vi "74_Vision_RC Servo_DC_Moto_2.vi"() -> ()   [LabVIEW 2018]
uses:
  <userlib>/KNR OS 4.0 LabVIEW Toolkit/Type Definition/Resource.ctl
  <userlib>/KNR OS 4.0 LabVIEW Toolkit/Type Definition/RC Servo Port.ctl
  <userlib>/KNR OS 4.0 LabVIEW Toolkit/Type Definition/DC Motor Port.ctl
panel:
  out "area":dbl
  out "RC Pulse Width (uS)":u16[](array[numeric])
  out "Image Out":T1(plugin-control)
  in  "stop":bool
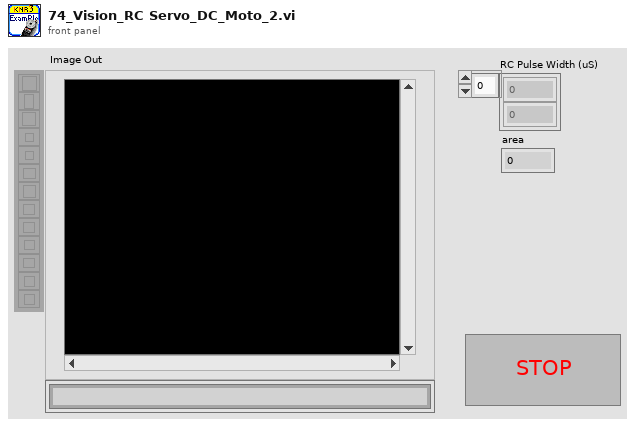
[diagram p1: front panel]
types:
  T1 = typedef "IMAQ Image.ctl" = refnum<image>
  T2 = typedef "DC Motor Port.ctl" = u16
  T3 = typedef "RC Servo Port.ctl" = u16
  T4 = typedef "Resource.ctl" = enum16{"KNRm_DDRC", "KNRm_DDDD", "KNRm_DDDR", "KNRm_DDDC", "KNR", "KNRm_neww"}
  T5 = typedef "KNR3 Reference.ctl" = cluster{"FPGA Session":refnum<class "FPGA Interface Base.lvclass">, "Resource":T4}
  T6 = cluster{"Left":dbl, "Top":dbl, "Right":dbl, "Bottom":dbl}
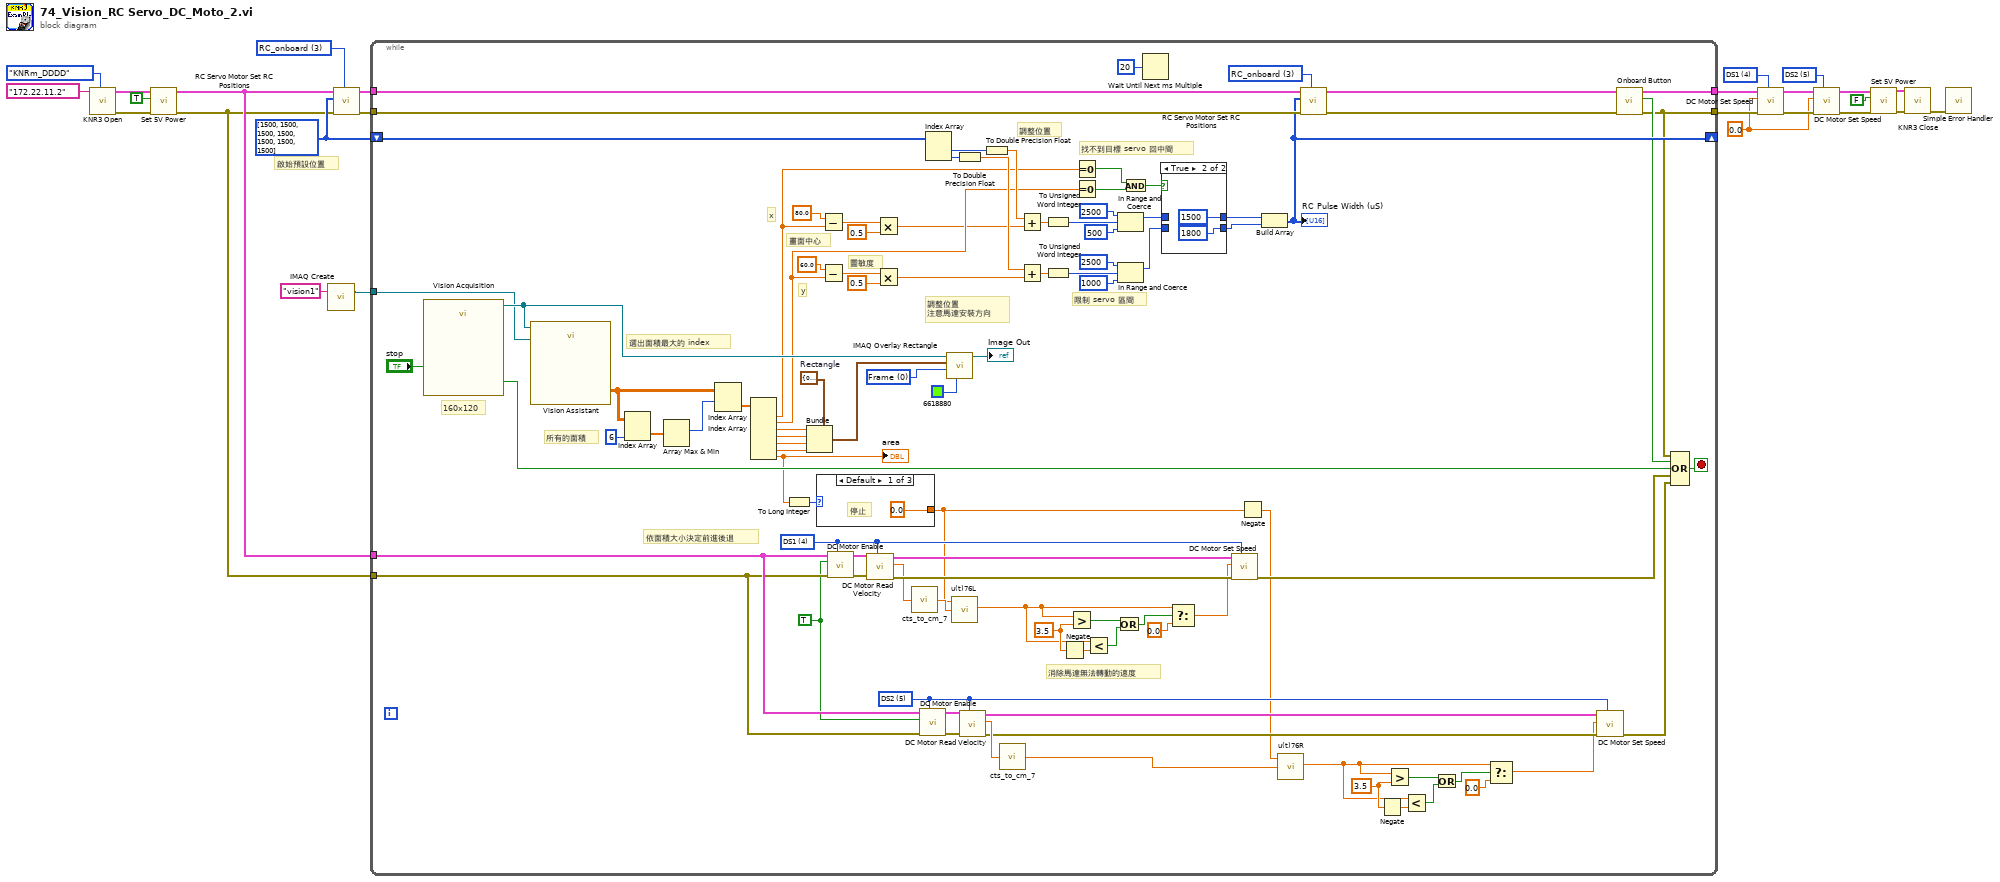
[diagram p0: block diagram]
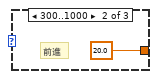
[diagram p2: hidden frame]
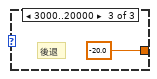
[diagram p3: hidden frame]
diagram:
  w1 = T2 5 items=["DS1"=4, "DS2"=5, "DS3"=6, "DS4"=7] ("Port (DS1)")
  w2 = T2 4 items=["DS1"=4, "DS2"=5, "DS3"=6, "DS4"=7] ("Port (DS1)")
  w3 = 0.0 ("Speed (+-100%)")
  w13 = u16[] [1500, 1500, 1500, 1500, 1500, 1500, 1500] ("RC Pulse Width (1500 uS)")
  w16 = T3 3 items=["RC_onboard"=3, "RC_box"=9] ("Port (RC_onboard)")
  # "啟始預設位置"
  n1 = call <userlib>:"KNR3 Open.vi"("Resource"=Resource."KNRm_DDDD", "IP"="172.22.11.2") -> ("error out"=w22:errorcluster, "KNR out"=w23:T5)  [unwired: 8 in]
  n2 = call <userlib>:"Set 5V Power.vi"("error in (no error)"=w22, "5V Power(T)"=TRUE ("5V Power"), "KNR in"=w23) -> ("error out"=w11:errorcluster, "KNR out"=w12:T5)  [unwired: 7 in]
  n3 = call "IMAQ Create"("Image Name"="vision1") -> ("New Image"=w14:T1)  [unwired: 4 in, 1 out]
  n4 = call <userlib>:"RC Servo Motor Set RC Positions.vi"("Port (RC_onboard)"=w16, "RC Pulse Width (1500 uS)"=w13, "KNR in"=w12) -> ("KNR out"=w17:T5)  [unwired: 7 in, 1 out]
  n5 = while {
    tunnel: w17 -> [w120]
    tunnel: [w43] -> w10
    tunnel: w11 -> [w118]
    tunnel: [w41] -> w9
    tunnel: w14 -> [w100]
    shift-right: [w84] -> _
    shift-left: w13 -> [w87]
    tunnel: w12 -> [w50]
    tunnel: w11 -> [w49]
    stop <- w117 stop-if-true
    w28 = 3.5
    w36 = 3.5
    w47 = u32 0 items=["Frame", "Fill", "Highlight"] ("Drawing Mode (Frame)")
    w53 = T2 5 items=["DS1"=4, "DS2"=5, "DS3"=6, "DS4"=7] ("Port 2")
    w44 = TRUE ("Enable Motor(F)")
    w66 = T2 4 items=["DS1"=4, "DS2"=5, "DS3"=6, "DS4"=7] ("Port 2")
    w113 = T6 {"Left"=0.0, "Top"=0.0, "Right"=0.0, "Bottom"=0.0}  # Rectangle
    w115 = T3 3 items=["RC_onboard"=3, "RC_box"=9] ("RC Motor")
    # "調整位置\n注意馬達安裝方向"
    # "依面積大小決定前進後退"
    # "消除馬達無法轉動的速度"
    # "調整位置"
    # "靈敏度"
    # "所有的面積"
    # "畫面中心"
    # "限制 servo 區間"
    # "找不到目標 servo 回中間"
    # "y"
    # "x"
    # "160x120"
    # "選出面積最大的 index"
    n6 = call "Vision Acquisition"("Stop (F)"="stop") -> ("Image Out"=w105:T1, "Stopped"=w98:bool)  [unwired: 24 in, 1 out]
    n7 = call "Vision Assistant"("Image In"=w105, "Image Dst"=w100) -> ("Particle Measurements (Pixels) (Particle Analysis 1)"=w104:dbl[][])  [unwired: 22 in, 3 out]
    n8 = Index Array "Index Array"(array=w104, index (col)=6 ("disabled index (col)")) -> (element=w103:dbl[])  [unwired: 1 in]
    n9 = Array Max & Min(array=w103) -> (max index (indices)=w102:i32)  [unwired: 3 out]
    n10 = Index Array "Index Array"(array=w104, index (row)=w102) -> (element=w114:dbl[])  [unwired: 1 in]
    n11 = Index Array "Index Array"(array=w114) -> (element #1=w77:dbl, element #2=w76:dbl, element #3=w112:dbl, element #4=w111:dbl, element #5=w110:dbl, element #6=w109:dbl, element #7=w60:dbl)  [unwired: 7 in]
    "area" <- w60
    n12 = To Long Integer(number=w60) -> (32bit integer=w46:i32)
    n13 = Bundle "Bundle"(cluster=w113, "Left"=w112, "Top"=w111, "Right"=w110, "Bottom"=w109) -> (w108:T6)
    n14 = case shown="Default" w46 {
      tunnel: [0.0 20.0 -20.0] -> w40
      frame Default {
        # "停止"
      }
      frame 300..1000 {
        # "前進"
      }
      frame 3000..20000 {
        # "後退"
      }
    }
    n15 = Subtract(x=80.0 ("y"), y=w77) -> (x-y=w94:dbl)
    n16 = Subtract(x=60.0 ("y"), y=w76) -> (x-y=w95:dbl)
    n17 = call <userlib>:"DC Motor Enable.vi"("Port (DS1)"=w66, "error in (no error)"=w49, "Enable Motor(F)"=w44, "KNR in"=w50) -> ("error out"=w62:errorcluster, "KNR out"=w61:T5)  [unwired: 6 in]
    n18 = call <userlib>:"DC Motor Read Velocity.vi"("Port (DS1)"=w66, "error in (no error)"=w62, "KNR in"=w61) -> ("error out"=w65:errorcluster, "Velocity (cts/sec)"=w63:dbl, "KNR out"=w64:T5)  [unwired: 6 in]
    n19 = Multiply(x=w94, y=0.5) -> (x*y=w75:dbl)
    n20 = Multiply(x=w95, y=0.5) -> (x*y=w74:dbl)
    n21 = call "cts_to_cm_7.vi"("cts"=w63) -> ("cm"=w45:dbl)
    n22 = call <userlib>:"DC Motor Enable.vi"("Port (DS1)"=w53, "error in (no error)"=w49, "Enable Motor(F)"=w44, "KNR in"=w50) -> ("error out"=w57:errorcluster, "KNR out"=w58:T5)  [unwired: 6 in]
    n23 = Index Array "Index Array"(array=w87) -> (element #1=w86:u16, element #2=w85:u16)  [unwired: 2 in]
    n24 = call "IMAQ Overlay Rectangle"("Color"=u32 6618880, "Drawing Mode (Frame)"=w47, "Rectangle"=w108, "Image"=w105) -> ("Image Out"=→"Image Out":T1)  [unwired: 6 in, 1 out]
    n25 = call "u(t)76L.vi"("Velocity"=w45, "Desire Velosity"=w40) -> ("u(t)"=w34:dbl)  [unwired: 6 in]
    n26 = To Double Precision Float(number=w85) -> (double precision float=w78:dbl)
    n27 = call <userlib>:"DC Motor Read Velocity.vi"("Port (DS1)"=w53, "error in (no error)"=w57, "KNR in"=w58) -> ("error out"=w54:errorcluster, "Velocity (cts/sec)"=w56:dbl, "KNR out"=w55:T5)  [unwired: 6 in]
    n28 = To Double Precision Float(number=w86) -> (double precision float=w79:dbl)
    n29 = call "cts_to_cm_7.vi"("cts"=w56) -> ("cm"=w59:dbl)
    n30 = Add(x=w79, y=w75) -> (x+y=w96:dbl)
    n31 = Add(x=w78, y=w74) -> (x+y=w97:dbl)
    n32 = To Unsigned Word Integer(number=w96) -> (unsigned 16bit integer=w81:u16)
    n33 = To Unsigned Word Integer(number=w97) -> (unsigned 16bit integer=w80:u16)
    n34 = Negate(x=w36) -> (-x=w35:dbl)
    n35 = Greater?(x=w34, y=w36) -> (0:w33:bool)
    n36 = Equal To 0?(x=w77) -> (x = 0?=w71:bool)
    n37 = Equal To 0?(x=w76) -> (x = 0?=w72:bool)
    n38 = Less?(x=w34, y=w35) -> (x < y?=w32:bool)
    n39 = Or(x=w33, y=w32) -> (x .or. y?=w37:bool)
    n40 = In Range and Coerce(upper limit=u16 2500, x=w81, lower limit=u16 500) -> (coerced(x)=w70:u16)  [unwired: 1 out]
    n41 = In Range and Coerce(upper limit=u16 2500, x=w80, lower limit=u16 1000) -> (coerced(x)=w69:u16)  [unwired: 1 out]
    n42 = And(x=w71, y=w72) -> (x .and. y?=w73:bool)
    n43 = Wait Until Next ms Multiple(millisecond multiple=u32 20) -> ()  [unwired: 1 out]
    n44 = case shown="True" w73 {
      tunnel: w70 -> [w125 _]
      tunnel: w69 -> [w124 _]
      tunnel: [w125 u16 1500] -> w68
      tunnel: [w124 u16 1800] -> w67
      frame False {
      }
      frame True {
      }
    }
    n45 = Select(t=w34, s=w37, f=0.0) -> (s? t:f=w39:dbl)
    n46 = call <userlib>:"DC Motor Set Speed.vi"("Port (DS1)"=w66, "error in (no error)"=w65, "Speed (+-100%)"=w39, "KNR in"=w64) -> ("error out"=w52:errorcluster)  [unwired: 6 in, 1 out]
    n47 = Negate(x=w40) -> (-x=w48:dbl)
    n48 = Build Array "Build Array"(w68, w67) -> (w84:u16[])
    "RC Pulse Width (uS)" <- w84
    n49 = call "u(t)76R.vi"("Desire Velosity"=w48, "Velocity"=w59) -> ("u(t)"=w25:dbl)  [unwired: 5 in]
    n50 = call <userlib>:"RC Servo Motor Set RC Positions.vi"("Port (RC_onboard)"=w115, "error in (no error)"=w118, "RC Pulse Width (1500 uS)"=w84, "KNR in"=w120) -> ("error out"=w41:errorcluster, "KNR out"=w119:T5)  [unwired: 6 in]
    n51 = Negate(x=w28) -> (-x=w29:dbl)
    n52 = Greater?(x=w25, y=w28) -> (0:w30:bool)
    n53 = Less?(x=w25, y=w29) -> (x < y?=w31:bool)
    n54 = Or(x=w30, y=w31) -> (x .or. y?=w27:bool)
    n55 = Select(t=w25, s=w27, f=0.0) -> (s? t:f=w24:dbl)
    n56 = call <userlib>:"DC Motor Set Speed.vi"("Port (DS1)"=w53, "error in (no error)"=w54, "Speed (+-100%)"=w24, "KNR in"=w55) -> ("error out"=w51:errorcluster)  [unwired: 6 in, 1 out]
    n57 = call <userlib>:"Onboard Button.vi"("KNR in"=w119) -> ("value"=w42:bool, "KNR out"=w43:T5)  [unwired: 8 in, 1 out]
    n58 = Compound Arithmetic op=OR(w41, w42, w98, w52, w51) -> (w117:bool)
  }
  n59 = call <userlib>:"DC Motor Set Speed.vi"("Port (DS1)"=w2, "Speed (+-100%)"=w3, "KNR in"=w10) -> ("KNR out"=w5:T5)  [unwired: 7 in, 1 out]
  n60 = call <userlib>:"DC Motor Set Speed.vi"("Port (DS1)"=w1, "Speed (+-100%)"=w3, "KNR in"=w5) -> ("KNR out"=w4:T5)  [unwired: 7 in, 1 out]
  n61 = call <userlib>:"Set 5V Power.vi"("error in (no error)"=w9, "5V Power(T)"=FALSE, "KNR in"=w4) -> ("error out"=w7:errorcluster, "KNR out"=w8:T5)  [unwired: 7 in]
  n62 = call <userlib>:"KNR3 Close.vi"("error in (no error)"=w7, "KNR in"=w8) -> ("error out"=w21:errorcluster)  [unwired: 9 in]
  n63 = call <vilib>:"Simple Error Handler.vi"("error in (no error)"=w21) -> ()  [unwired: 4 in, 5 out]
